vi "GetPanePositionString.vi"(8 "error in (no error)":errorcluster, 10 "PaneRef":refnum<vi>, 11 "PentaPanesGUI in":refnum<class "PentaPanes.lvclass">) -> (0 "error out":errorcluster, 1 "Label.Text":string, 2 "Pos String":string, 3 "PentaPanesGUI out":refnum<class "PentaPanes.lvclass">)   [LabVIEW 2022 SP3, in "PentaPanesLibrary.lvlib" / "PentaPanes.lvclass"]
doc: "This VI reads the Pane's position string and Label.\n\nPaneRef - A reference to the pane. \nPos String - Outputs a position string (\"Top\", \"Left\", \"Right\", \"Bottom\").\nLabel.Text - Outputs The Label of the pane."
uses:
  PentaPanes.lvclass
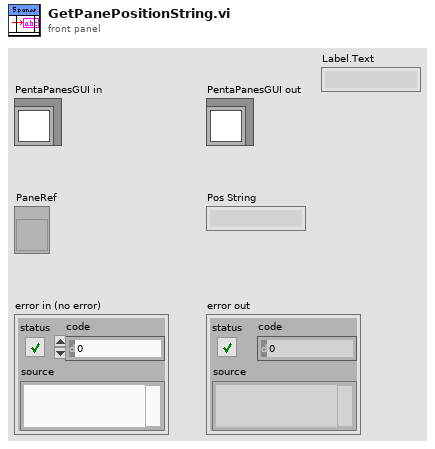
[diagram p1: front panel]
types:
  T1 = typedef "PentaPanesLibrary.lvlib/PentaPanes.lvclass/PanesCluster.ctl" = cluster{"Top Pane":refnum<vi>, "Left Pane":refnum<vi>, "Center Pane":refnum<vi>, "Right Pane":refnum<vi>, "Bottom Pane":refnum<vi>}
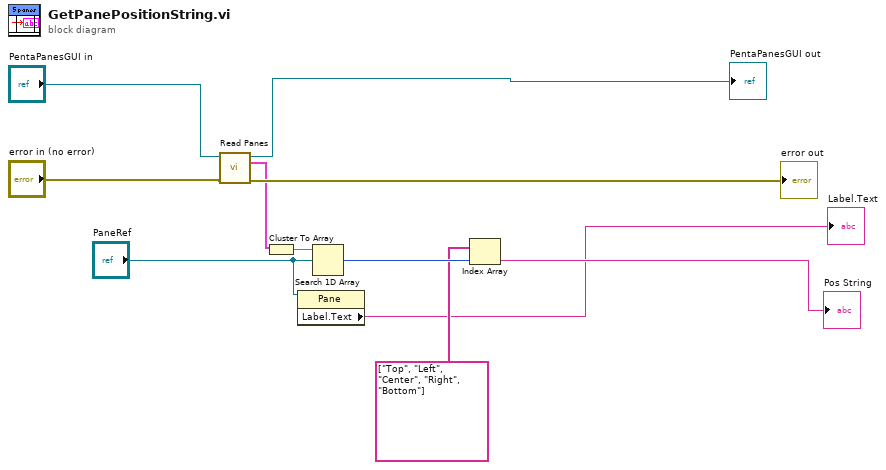
[diagram p0: block diagram]
diagram:
  n1 = call-dynamic "Read Panes.vi"("error in (no error)"="error in (no error)", "PentaPanesGUI in"="PentaPanesGUI in") -> ("error out"=→"error out":errorcluster, "Panes"=w5:T1, "PentaPanesGUI out"=→"PentaPanesGUI out":refnum<class "PentaPanes.lvclass">)  [unwired: 7 in]
  n2 = Cluster To Array(cluster=w5) -> (array=w6:refnum<vi>[])
  n3 = property class="Pane"(reference="PaneRef") -> ("Label.Text"=→"Label.Text":string)  [unwired: 1 in, 2 out]
  n4 = Search 1D Array(1D array=w6, element="PaneRef") -> (index of element=w10:i32)  [unwired: 1 in]
  n5 = Index Array(array=string[] ["Top", "Left", "Center", "Right", "Bottom"], index=w10) -> (element=→"Pos String":string)
